vi "sub FM0decodeGet16.vi"(10 "threshold":i32=3, 11 "RN16 waveform":i16[](array[numeric])) -> (3 "RN16 array":i32[](array[numeric]))   [LabVIEW 2015]
doc: "This example shows how the Write to Text File and Read from Text File functions operate using different options."
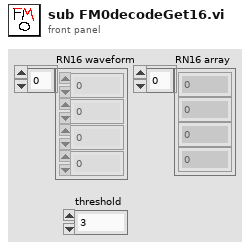
[diagram p1: front panel]
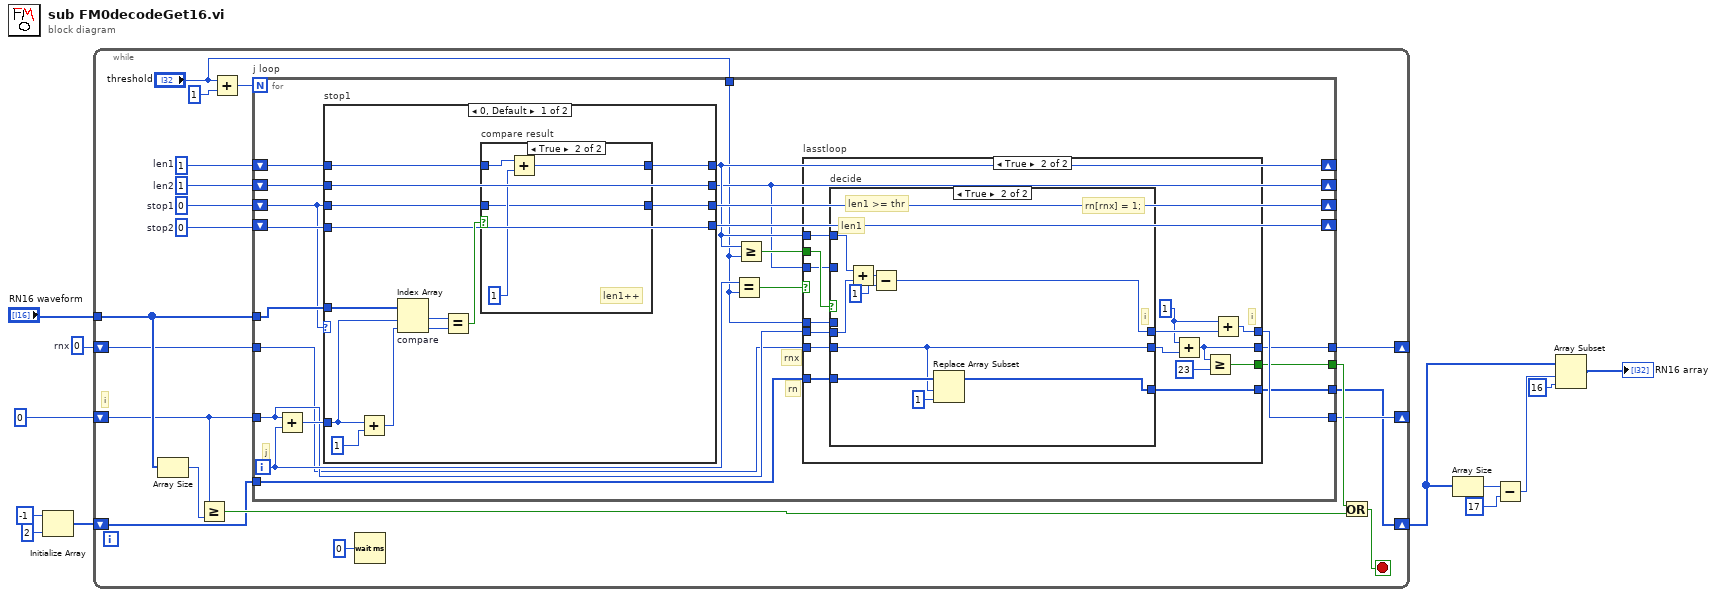
[diagram p0: block diagram]
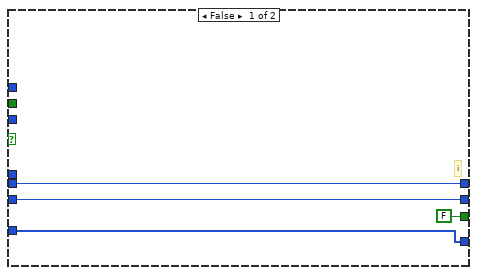
[diagram p2: hidden frame]
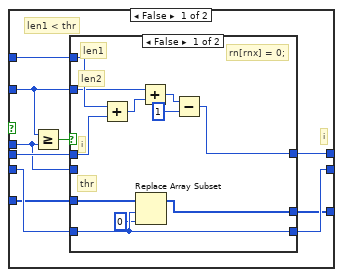
[diagram p3: hidden frame]
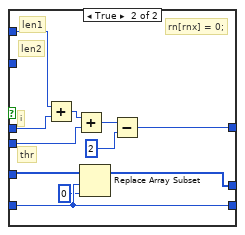
[diagram p4: hidden frame]
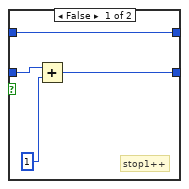
[diagram p5: hidden frame]
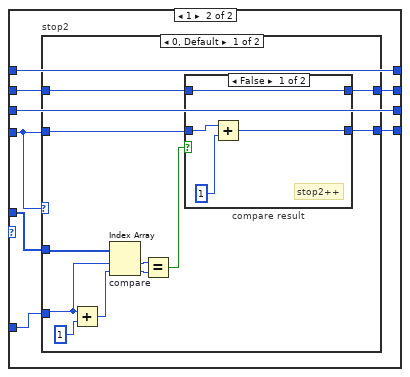
[diagram p6: hidden frame]
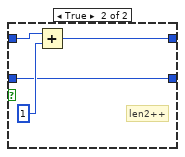
[diagram p7: hidden frame]
diagram:
  w12 = 0  # rnx
  n1 = Initialize Array(-1 ("element"), 2 ("dimension size")) -> (w10:i32[])
  n2 = while {
    tunnel: "RN16 waveform" -> [w27]
    shift-right: [w15] -> _
    shift-left: 0 -> [w16]
    shift-right: [w18] -> _
    shift-left: w12 -> [w17]
    shift-right: [w13] -> w6
    shift-left: w10 -> [w14]
    stop <- w24 stop-if-true
    w31 = 0  # stop2
    w30 = 0  # stop1
    w29 = 1  # len2
    w28 = 1  # len1
    # "i"
    n3 = Array Size(array=w27) -> (size(s)=w26:i32)
    n4 = Greater Or Equal?(x=w16, y=w26) -> (x >= y?=w23:bool)
    n5 = Add(x="threshold", y=1) -> (x+y=w20:i32)
    n6 = for "j loop" {
      N: w20 -> [_]
      tunnel: w27 -> [w48]
      shift-right: [w40] -> _
      shift-left: w28 -> [w52]
      shift-right: [w46] -> _
      shift-left: w30 -> [w47]
      shift-right: [w45] -> _
      shift-left: w31 -> [w50]
      shift-right: [w36] -> _
      shift-left: w29 -> [w51]
      tunnel: "threshold" -> [w34]
      tunnel: [w35] -> w25
      tunnel: w16 -> [w41]
      tunnel: [w39] -> w15
      tunnel: w17 -> [w38]
      tunnel: [w37] -> w18
      tunnel: w14 -> [w33]
      tunnel: [w32] -> w13
      i -> [w44]
      # "rn"
      # "rnx"
      # "j"
      n7 = Add(x=w41, y=w44) -> (x+y=w49:i32)
      n8 = case "stop1" shown="0, Default" w47 {
        tunnel: w52 -> [w118 w141]
        tunnel: w51 -> [w114 w136]
        tunnel: w50 -> [w113 w138]
        tunnel: w49 -> [w124 w134]
        tunnel: w48 -> [w122 w139]
        tunnel: [w117 w141] -> w40
        tunnel: w47 -> [w116 w140]
        tunnel: [w115 w140] -> w46
        tunnel: [w113 w137] -> w45
        tunnel: [w114 w135] -> w36
        frame 0, Default {
          n9 = Add(x=w124, y=1) -> (x+y=w125:i32)
          n10 = Index Array "compare"(array=w122, index #1=w124, index #2=w125) -> (element #1=w120:i16, element #2=w121:i16)
          n11 = Equal?(x=w120, y=w121) -> (x = y?=w119:bool)
          n12 = case "compare result" shown="True" w119 {
            tunnel: w118 -> [w129 w133]
            tunnel: [w129 w132] -> w117
            tunnel: w116 -> [w127 w130]
            tunnel: [w128 w130] -> w115
            frame False {
              # "stop1++"
              n13 = Add(x=w127, y=1) -> (x+y=w128:i32)
            }
            frame True {
              # "len1++"
              n14 = Add(x=w133, y=1) -> (x+y=w132:i32)
            }
          }
        }
        frame 1 {
          n15 = case "stop2" shown="0, Default" w138 {
            tunnel: w139 -> [w149 _]
            tunnel: w138 -> [w148 w161]
            tunnel: [w147 w161] -> w137
            tunnel: w136 -> [w146 w162]
            tunnel: [w145 w162] -> w135
            tunnel: w134 -> [w142 _]
            frame 0, Default {
              n16 = Add(x=w142, y=1) -> (x+y=w150:i32)
              n17 = Index Array "compare"(array=w149, index #1=w142, index #2=w150) -> (element #1=w152:i16, element #2=w151:i16)
              n18 = Equal?(x=w152, y=w151) -> (x = y?=w143:bool)
              n19 = case "compare result" shown="False" w143 {
                tunnel: w146 -> [w156 w160]
                tunnel: [w156 w159] -> w145
                tunnel: w148 -> [w154 w157]
                tunnel: [w155 w157] -> w147
                frame False {
                  # "stop2++"
                  n20 = Add(x=w154, y=1) -> (x+y=w155:i32)
                }
                frame True {
                  # "len2++"
                  n21 = Add(x=w160, y=1) -> (x+y=w159:i32)
                }
              }
            }
            frame 1 {
            }
          }
        }
      }
      n22 = Equal?(x=w44, y=w34) -> (x = y?=w43:bool)
      n23 = Greater Or Equal?(x=w40, y=w34) -> (x >= y?=w42:bool)
      n24 = case "lasstloop" shown="True" w43 {
        tunnel: w42 -> [_ w69]
        tunnel: w41 -> [w56 w71]
        tunnel: w40 -> [_ w70]
        tunnel: [w56 w62] -> w39
        tunnel: w38 -> [w55 w60]
        tunnel: [w55 w67] -> w37
        tunnel: w36 -> [_ w68]
        tunnel: [FALSE w65] -> w35
        tunnel: w34 -> [_ w64]
        tunnel: w33 -> [w53 w58]
        tunnel: [w53 w57] -> w32
        frame False {
          # "i"
        }
        frame True {
          w61 = 1 ("y")
          # "i"
          n25 = case "decide" shown="True" w69 {
            tunnel: w71 -> [w81 w111]
            tunnel: w70 -> [w77 w112]
            tunnel: [w76 w109] -> w63
            tunnel: w68 -> [w79 _]
            tunnel: w64 -> [w78 _]
            tunnel: [w74 w105] -> w59
            tunnel: w60 -> [w75 w105]
            tunnel: w58 -> [w73 w107]
            tunnel: [w72 w106] -> w57
            frame False {
              # "i"
              # "len1 < thr"
              n26 = Greater Or Equal?(x=w79, y=w78) -> (x >= y?=w80:bool)
              n27 = case shown="False" w80 {
                tunnel: w79 -> [w89 _]
                tunnel: w81 -> [w91 w102]
                tunnel: w78 -> [_ w100]
                tunnel: w77 -> [w92 w103]
                tunnel: [w86 w97] -> w76
                tunnel: [w84 w94] -> w74
                tunnel: w75 -> [w84 w94]
                tunnel: w73 -> [w85 w96]
                tunnel: [w82 w95] -> w72
                frame False {
                  # "rn[rnx] = 0;"
                  # "thr"
                  # "len2"
                  # "i"
                  # "len1"
                  n28 = Add(x=w92, y=w91) -> (x+y=w90:i32)
                  n29 = Replace Array Subset(array=w85, new element=0 ("new element/subarray"), index=w84) -> (w82:i32[])
                  n30 = Add(x=w89, y=w90) -> (x+y=w88:i32)
                  n31 = Subtract(x=w88, y=1) -> (x-y=w86:i32)
                }
                frame True {
                  # "rn[rnx] = 0;"
                  # "len2"
                  # "thr"
                  # "i"
                  # "len1"
                  n32 = Add(x=w103, y=w102) -> (x+y=w101:i32)
                  n33 = Add(x=w101, y=w100) -> (x+y=w99:i32)
                  n34 = Replace Array Subset(array=w96, new element=0 ("new element/subarray"), index=w94) -> (w95:i32[])
                  n35 = Subtract(x=w99, y=2) -> (x-y=w97:i32)
                }
              }
            }
            frame True {
              # "rn[rnx] = 1;"
              # "len1"
              # "i"
              # "len1 >= thr"
              n36 = Add(x=w112, y=w111) -> (x+y=w110:i32)
              n37 = Subtract(x=w110, y=1) -> (x-y=w109:i32)
              n38 = Replace Array Subset(array=w107, new element=1 ("new element/subarray"), index=w105) -> (w106:i32[])
            }
          }
          n39 = Add(x=w61, y=w59) -> (x+y=w67:i32)
          n40 = Greater Or Equal?(x=w67, y=23) -> (x >= y?=w65:bool)
          n41 = Add(x=w61, y=w63) -> (x+y=w62:i32)
        }
      }
    }
    n42 = Wait (ms)(milliseconds to wait=u32 0) -> ()  [unwired: 1 out]
    n43 = Or(x=w25, y=w23) -> (x .or. y?=w24:bool)
  }
  n44 = Array Size(array=w6) -> (size(s)=w5:i32)
  n45 = Subtract(x=w5, y=17) -> (x-y=w3:i32)
  n46 = Array Subset(array=w6, index=w3, length=16) -> (→"RN16 array":i32[])
